vi "Is_TestDataInSpec- 单值-四舍五入-输入为量测内容.vi"(3 "量测内容":T1={"点位名称"="", "选择螺丝供料机"=enum."1号供料机", "螺丝型号"=enum."一字M3*8", "点位坐标(图纸)"={"X"=0.0, "Y"=0.0, "Z"=0.005}, "点位坐标(实际)"={"X"=0.0, "Y"=0.0, "Z"=1.0}, "锁附时机械手角度"=enum."0度"}, 5 "数值":dbl format="%#_13g") -> (0 "进位舍位后值":dbl format="%#_13g", 1 "在规格内":bool)   [LabVIEW 2014]
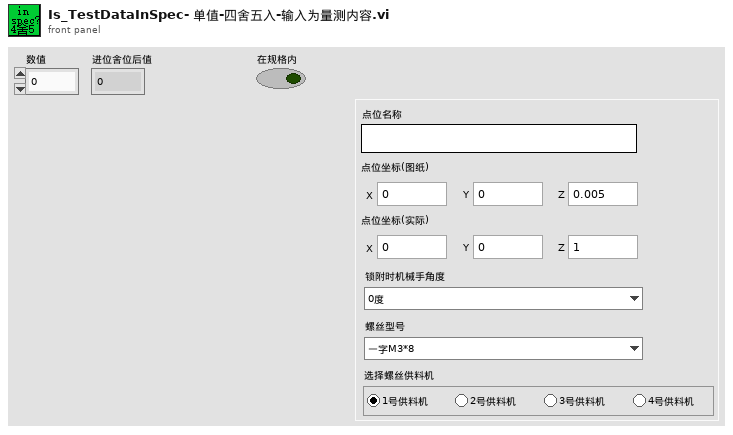
[diagram p1: front panel]
types:
  T1 = typedef "锁附点位信息.ctl" = cluster{"点位名称":string, "选择螺丝供料机":enum32{"1号供料机", "2号供料机", "3号供料机", "4号供料机"}, "螺丝型号":T2, "点位坐标(图纸)":T3, "点位坐标(实际)":T3, "锁附时机械手角度":T4}
  T2 = typedef "螺丝型号.ctl" = enum16{"不供料", "一字M3*8", "一字M3*12", "一字M5*8", "一字M5*12", "十字M3*8", "十字M3*12", "十字M5*8", "十字M5*12"}
  T3 = typedef "锁附点位坐标XYZ.ctl" = cluster{"X":dbl, "Y":dbl, "Z":dbl}
  T4 = typedef "锁附时机械手角度.ctl" = enum16{"0度", "90度", "180度", "270度"}
  T5 = typedef "TestThreshold.ctl" = cluster{"下限":dbl, "上限":dbl}
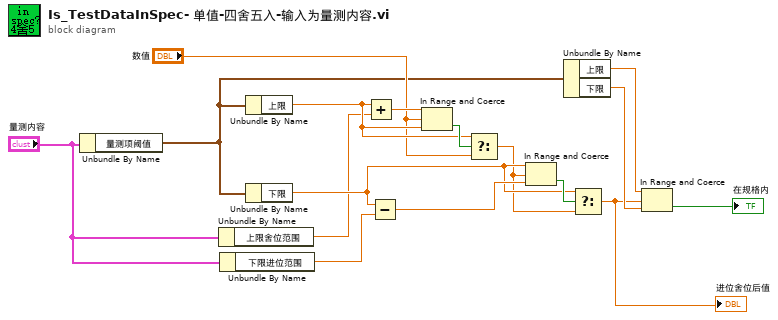
[diagram p0: block diagram]
diagram:
  n1 = Unbundle By Name("量测内容") -> ("量测项阈值"=w4:T5)
  n2 = Unbundle By Name("量测内容") -> ("上限舍位范围"=w2:dbl)
  n3 = Unbundle By Name("量测内容") -> ("下限进位范围"=w1:dbl)
  n4 = Unbundle By Name(w4) -> ("上限"=w14:dbl)
  n5 = Unbundle By Name(w4) -> ("下限"=w9:dbl)
  n6 = Add(x=w14, y=w2) -> (x+y=w16:dbl)
  n7 = Subtract(x=w9, y=w1) -> (x-y=w12:dbl)
  n8 = In Range and Coerce(upper limit=w16, x="数值", lower limit=w14) -> (In Range?=w15:bool)  [unwired: 1 out]
  n9 = Select(t=w14, s=w15, f="数值") -> (s? t:f=w8:dbl)
  n10 = In Range and Coerce(upper limit=w9, x=w8, lower limit=w12) -> (In Range?=w13:bool)  [unwired: 1 out]
  n11 = Unbundle By Name(w4) -> ("上限"=w10:dbl, "下限"=w11:dbl)
  n12 = Select(t=w9, s=w13, f=w8) -> (s? t:f=w6:dbl)
  "进位舍位后值" <- w6
  n13 = In Range and Coerce(upper limit=w10, x=w6, lower limit=w11) -> (In Range?=→"在规格内":bool)  [unwired: 1 out]
